vi "SCPI.vi"(4 "error in":T13, 7 "Command":string) -> (0 "error out":T13, 3 "Response":T11)   [LabVIEW 2018]
uses:
  MOKO_LabViewLibrary/MokoLowLevel/MokoLowLovelControl/MLLC_Error.ctl
  MOKO_LabViewLibrary/MokoLowLevel/MokoLowLovelControl/MLLC_Mode.ctl
  MOKO_LabViewLibrary/MokoLowLevel/MokoLowLovelControl/MLLC_Response.ctl
  MOKO_LabViewLibrary/MokoLowLevel/MokoLowLovelControl/MLLC_ConnectCluster.ctl
  MOKO_LabViewLibrary/MokoLowLevel/MokoLowLovelControl/MLLC_InterfaceType.ctl
  MOKO_LabViewLibrary/MokoLowLevel/MokoLowLovelControl/MLLC_OpenedSession.ctl
  MOKO_LabViewLibrary/MokoLowLevel/MokoLowLovelControl/MLLC_InterfaceSettings.ctl
  MOKO_LabViewLibrary/MokoLowLevel/MokoLowLovelControl/MLLC_InterfaceKind.ctl
  MOKO_LabViewLibrary/MokoLowLevel/MokoLowLovelControl/MLLC_DriverName.ctl
  MOKO_LabViewLibrary/MokoLowLevel/MokoLowLovelControl/MLLC_ErrorCode.ctl
  MOKO_LabViewLibrary/MokoLowLevel/MokoLowLovelControl/MLLC_ResponseInit.ctl
  MOKO_LabViewLibrary/MokoLowLevel/MokoLowLovelControl/MLLC_Request.ctl
panel:
  in  "Request":T1="*IDN?"
  in  "Response Init":T2="SCPI"
  in  "Error Code":T3=5450
  in  "Driver Name":T4="SCPI"
  in  "Settings":T10={"Saved Data"=variant, "Permanent data"={"Connect"={"InterfaceType"=enum."VISA", "OpenedSession"="COM1", "InterfaceSettings"={"Interface"=enum."Ethernet", "EOS 4 read"=enum."LF (\\n)", "EOS 4 write"=enum."LF (\\n)", "TMO, ms"=10000, "Sett"=variant(cluster{"Baud Rate":u32, "Data Bits":u16, "Parity":u16, "Stop Bits":u16, "Flow Control":u16, "Eho":bool} {"Baud Rate"=75, "Data Bits"=0, "Parity"=0, "Stop Bits"=0, "Flow Control"=0, "Eho"=FALSE})}}}}
  in  "Mode":T12=enum."Check"
  # "Example SCPI"
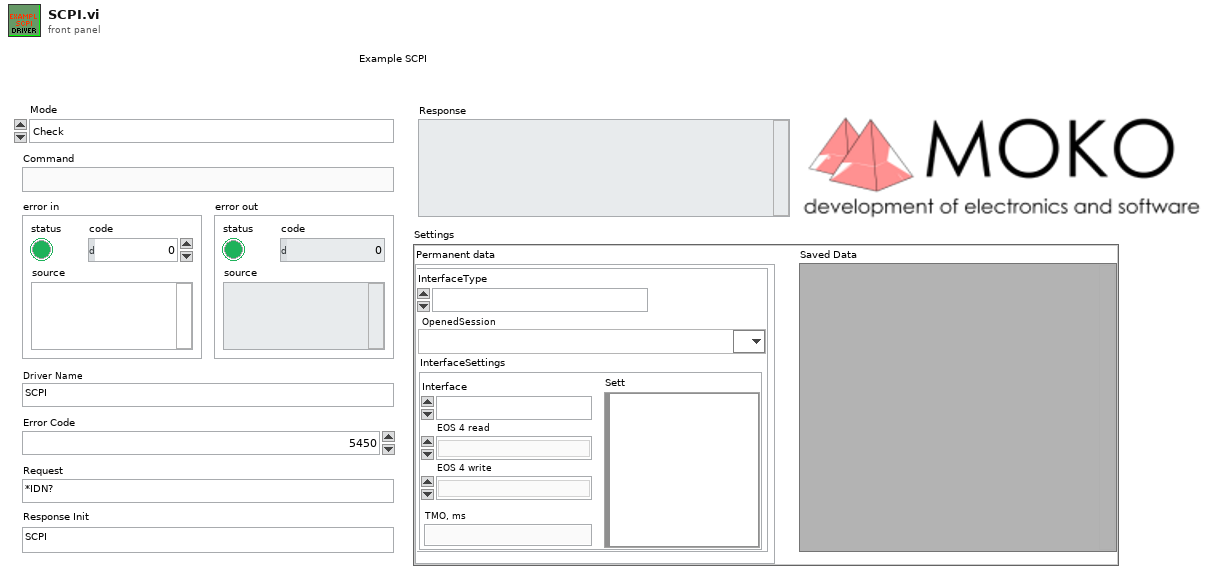
[diagram p1: front panel]
types:
  T1 = typedef "MLLC_Request.ctl" = string
  T2 = typedef "MLLC_ResponseInit.ctl" = string
  T3 = typedef "MLLC_ErrorCode.ctl" = u32
  T4 = typedef "MLLC_DriverName.ctl" = string
  T5 = typedef "MLLC_ConnectCluster.ctl" = cluster{"InterfaceType":T6, "OpenedSession":T7, "InterfaceSettings":T8}
  T6 = typedef "MLLC_InterfaceType.ctl" = enum16{"VISA", "Prologix USB-GPIB"}
  T7 = typedef "MLLC_OpenedSession.ctl" = refnum<visa-resource-name>
  T8 = typedef "MLLC_InterfaceSettings.ctl" = cluster{"Interface":T9, "EOS 4 read":enum16{"Default (=EOS 4 write)", "CR (\\r)", "LF (\\n)", "None"}, "EOS 4 write":enum16{"CR+LF (\\r\\n)", "CR (\\r)", "LF (\\n)", "None"}, "TMO, ms":i32, "Sett":variant}
  T9 = typedef "MLLC_InterfaceKind.ctl" = enum16{"RS232", "GPIB", "USB", "Ethernet", "another"}
  T10 = cluster{"Saved Data":variant, "Permanent data":cluster{"Connect":T5}}
  T11 = typedef "MLLC_Response.ctl" = string
  T12 = typedef "MLLC_Mode.ctl" = enum16{"get", "set", "close", "Init", "Check"}
  T13 = typedef "MLLC_Error.ctl" = errorcluster
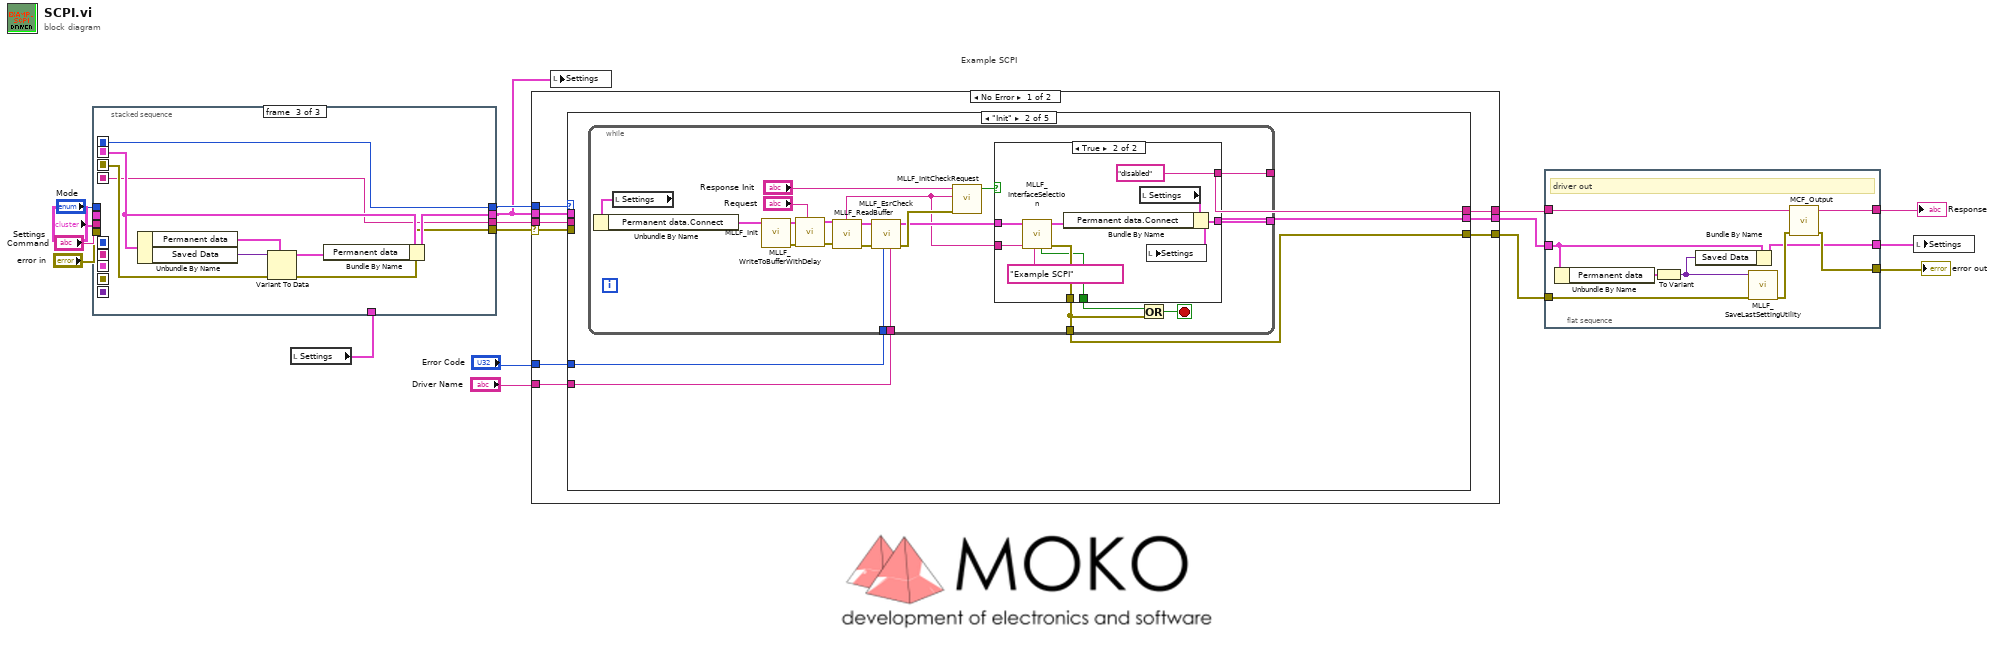
[diagram p0: block diagram]
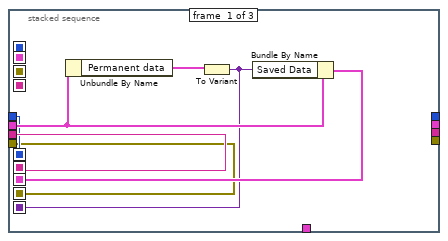
[diagram p2: hidden frame]
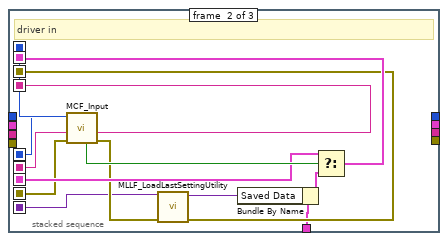
[diagram p3: hidden frame]
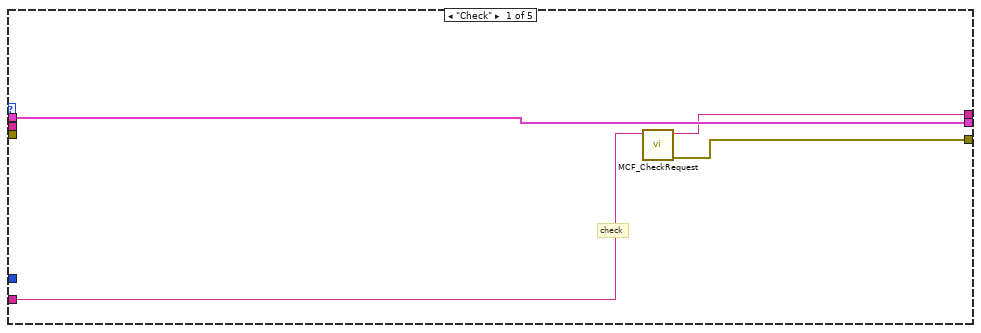
[diagram p4: hidden frame]
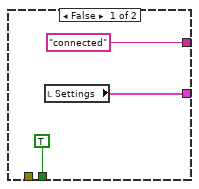
[diagram p5: hidden frame]
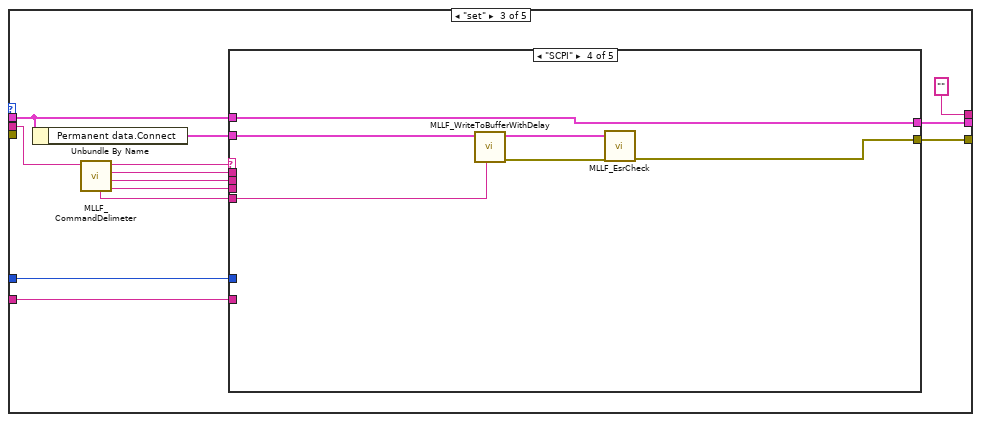
[diagram p6: hidden frame]
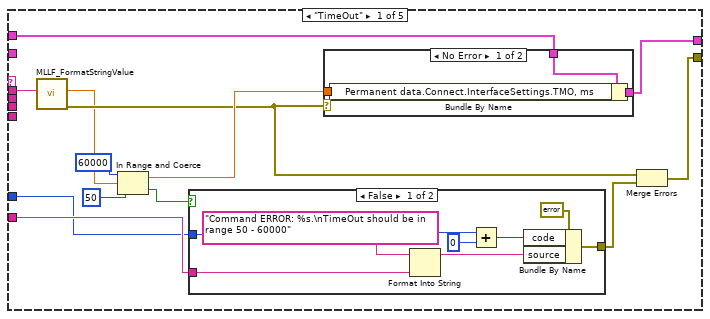
[diagram p7: hidden frame]
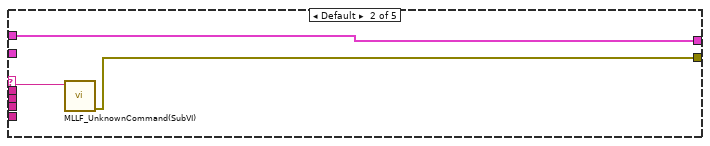
[diagram p10: hidden frame]
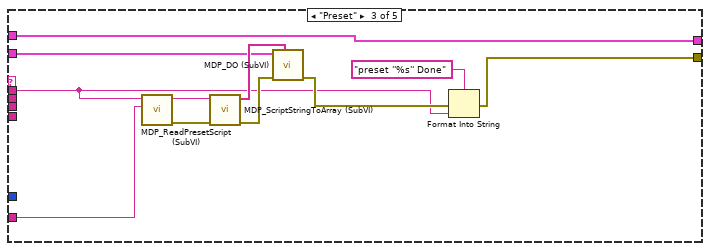
[diagram p11: hidden frame]
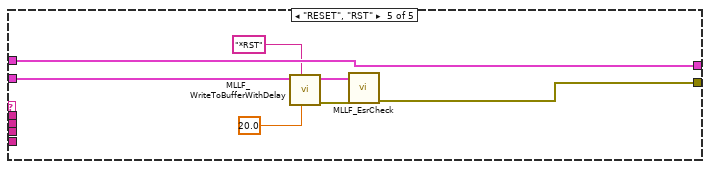
[diagram p12: hidden frame]
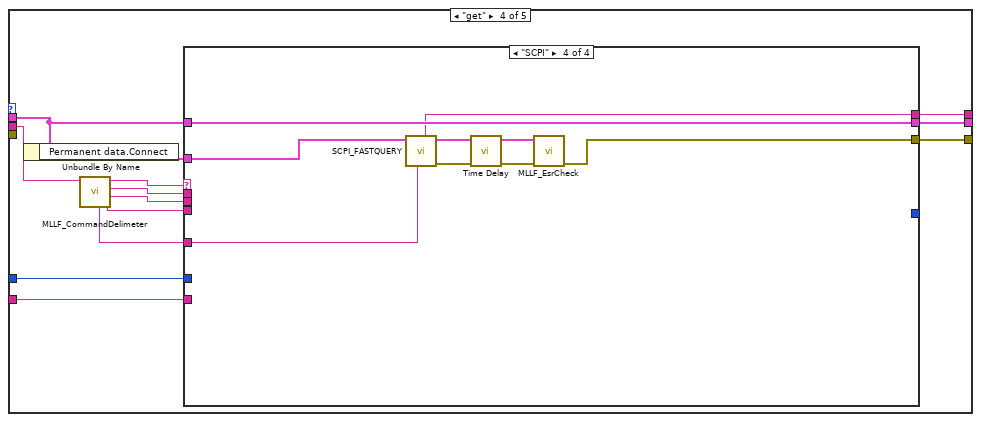
[diagram p13: hidden frame]
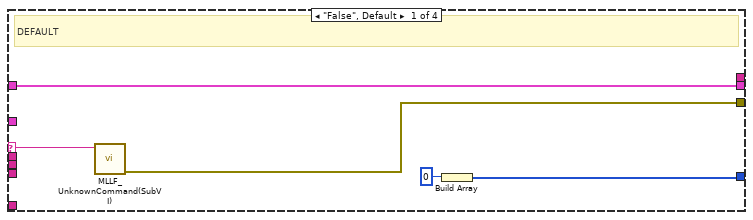
[diagram p14: hidden frame]
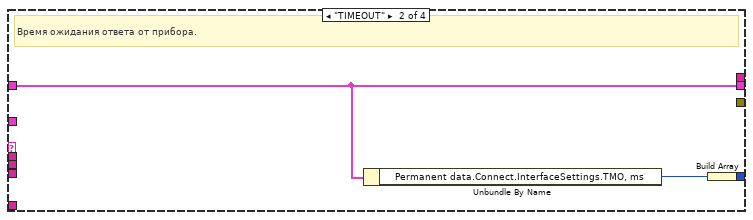
[diagram p15: hidden frame]
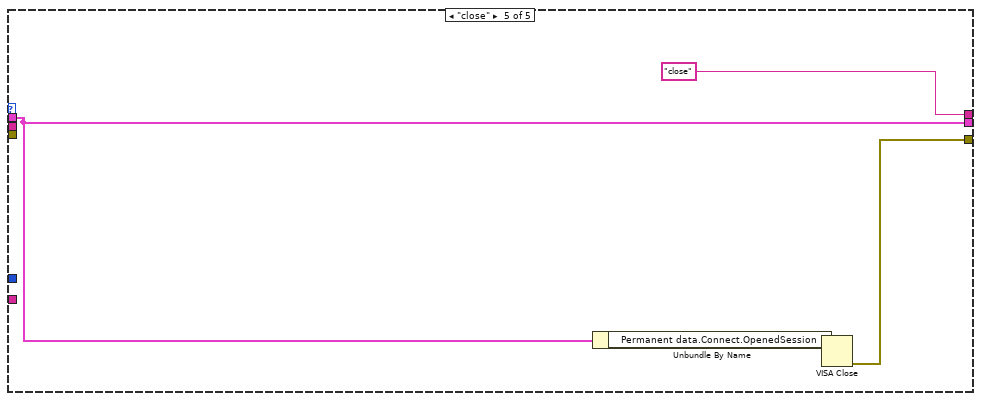
[diagram p17: hidden frame]
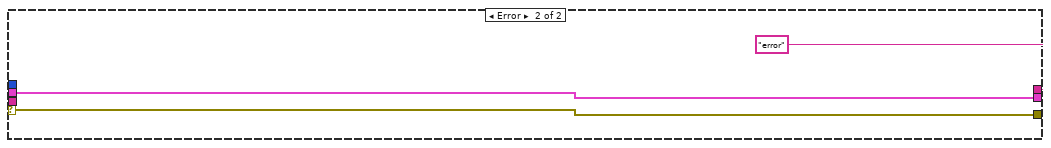
[diagram p18: hidden frame]
diagram:
  # "Example SCPI"
  n1 = local read "Settings"() -> (w7:T10)
  n2 = stacked-sequence {
    seq-local: [w20 _ _] -> [_ w36 _]
    seq-local: [w19 _ _] -> [_ w37 _]
    seq-local: [w22 _ _] -> [_ w32 _]
    seq-local: [w18 _ _] -> [_ w31 _]
    seq-local: [w21 _ _] -> [_ w27 _]
    seq-local: [_ w28 _] -> [_ _ w44]
    seq-local: [_ w38 _] -> [_ _ w41]
    seq-local: [_ w35 _] -> [_ _ w40]
    seq-local: [_ w34 _] -> [_ _ w45]
    tunnel: "Command" -> [w20 _ _]
    tunnel: "Mode" -> [w19 _ _]
    tunnel: "error in" -> [w18 _ _]
    tunnel: "Settings" -> [w23 _ _]
    tunnel: w7 -> [_ w26 _]
    tunnel: [_ _ w40] -> w9
    tunnel: [_ _ w43] -> w10
    tunnel: [_ _ w42] -> w8
    tunnel: [_ _ w41] -> w11
    frame #0 {
      n3 = Unbundle By Name(w23) -> ("Permanent data"=w24:cluster{"Connect":T5})
      n4 = To Variant(anything=w24) -> (Variant=w21:variant)
      n5 = Bundle By Name(cluster=w23, "Saved Data"=w21) -> (w22:T10)
    }
    frame #1 {
      # "driver in"
      n6 = call "MCF_Input.vi"("Error In"=w31, "Command in"=w36, "Mode in"=w37) -> ("Error Out"=w30:errorcluster, "Command out"=w35:string, "Mode out"=w38:T12, "Boolean"=w33:bool)  [unwired: 5 in]
      n7 = call "MLLF_LoadLastSettingUtility.vi"("Error In"=w30, "Save data in"=w27) -> ("Error Out"=w28:errorcluster, "Save data out"=w25:variant)  [unwired: 8 in]
      n8 = Bundle By Name(cluster=w26, "Saved Data"=w25) -> (w29:T10)
      n9 = Select(t=w32, s=w33, f=w29) -> (s? t:f=w34:T10)
    }
    frame #2 {
      n10 = Unbundle By Name(w45) -> ("Permanent data"=w46:cluster{"Connect":T5}, "Saved Data"=w39:variant)
      n11 = Variant To Data(error in=w44, type=w46, Variant=w39) -> (data=w47:cluster{"Connect":T5}, error out=w42:errorcluster)
      n12 = Bundle By Name(cluster=w45, "Permanent data"=w47) -> (w43:T10)
    }
  }
  n13 = case shown="No Error" w8 {
    selector: w8 -> [w52 w200]
    tunnel: [w54 w200] -> w4
    tunnel: w11 -> [w56 _]
    tunnel: [w55 "error" ("Output String")] -> w6
    tunnel: w9 -> [w53 _]
    tunnel: w10 -> [w49 w199]
    tunnel: "Error Code" -> [w51 _]
    tunnel: "Driver Name" -> [w50 _]
    tunnel: [w48 w199] -> w5
    frame No Error {
      n14 = case shown="\"Init\"" w56 {
        tunnel: [w58 w63 "" ("Output String") w168 "close" ("Output String")] -> w55
        tunnel: [w57 w62 w104 w170 w196] -> w54
        tunnel: w53 -> [_ _ w111 w176 _]
        tunnel: w52 -> [_ _ _ _ _]
        tunnel: w51 -> [_ w65 w110 w173 _]
        tunnel: w50 -> [w59 w64 w107 w172 _]
        tunnel: w49 -> [w60 _ w109 w175 w195]
        tunnel: [w60 w61 w108 w174 w195] -> w48
        frame "Check" {
          # "check"
          # "Проверка подленности пользователя в соответствии с протоколом MD5."
          n15 = call "MCF_CheckRequest.vi"("Driver Name"=w59) -> ("Error Out"=w57:errorcluster, "Output String"=w58:string)  [unwired: 9 in]
        }
        frame "Init" {
          # "Тут проходит инициализация оборудования"
          n16 = while {
            tunnel: [w79] -> w62
            tunnel: w65 -> [w72]
            tunnel: w64 -> [w71]
            tunnel: [w76] -> w63
            tunnel: [w77] -> w61
            stop <- w78 stop-if-true
            n17 = local read "Settings"() -> (w82:T10)
            n18 = Unbundle By Name(w82) -> ("Permanent data.Connect"=w74:T5)
            n19 = call "MLLF_Init.vi"("DriverConnect in"=w74) -> ("Error Out"=w84:errorcluster, "DriverConnect out"=w83:T5)  [unwired: 7 in]
            n20 = call "MLLF_WriteToBufferWithDelay.vi"("Command"="Request", "Error In"=w84, "DriverConnect in"=w83) -> ("Error Out"=w86:errorcluster, "DriverConnect out"=w85:T5)  [unwired: 7 in]
            n21 = call "MLLF_ReadBuffer.vi"("Error In"=w86, "DriverConnect in"=w85) -> ("Error Out"=w69:errorcluster, "DriverConnect out"=w70:T5, "String"=w66:string)  [unwired: 6 in]
            n22 = call "MLLF_EsrCheck.vi"("Name"=w71, "Error code"=w72, "error in"=w69, "DriverConnect in"=w70) -> ("error out"=w68:T13, "DriverConnect out"=w67:T5)  [unwired: 6 in]
            n23 = call "MLLF_InitCheckRequest.vi"("error in (no error)"=w68, "Answer"=w66, "Response Init"="Response Init") -> ("Design"=w73:bool)  [unwired: 5 in, 3 out]
            n24 = case shown="True" w73 {
              tunnel: w67 -> [_ w97]
              tunnel: [TRUE w91] -> w80
              tunnel: [_ w98] -> w79
              tunnel: [w88 w93] -> w77
              tunnel: ["connected" "disabled"] -> w76
              tunnel: w66 -> [_ w90]
              frame False {
                n25 = local read "Settings"() -> (w88:T10)
              }
              frame True {
                n26 = call "MLLF_InterfaceSelection.vi"("Driver Name"="Example SCPI" ("String"), "Answer:"=w90, "DriverConnect in"=w97) -> ("error out"=w98:T13, "DriverConnect out"=w95:T5, "stop init?"=w91:bool)  [unwired: 4 in, 2 out]
                n27 = local read "Settings"() -> (w94:T10)
                n28 = Bundle By Name(cluster=w94, "Permanent data.Connect"=w95) -> (w93:T10)
                n29 = local write "Settings"(w93) -> ()
              }
            }
            n30 = Or(x=w80, y=w79) -> (x .or. y?=w78:bool)
          }
        }
        frame "set" {
          # "Тут реализованы функции DriverSet"
          n31 = Unbundle By Name(w109) -> ("Permanent data.Connect"=w105:T5)
          n32 = call "MLLF_CommandDelimeter.vi"("command with param"=w111) -> ("param 3"=w100:string, "param 2"=w101:string, "param 1"=w102:string, "command"=w103:string, "Spit delimetre"=w99:string)  [unwired: 6 in]
          n33 = case shown="\"SCPI\"" w103 {
            selector: w103 -> [_ w138 _ _ _]
            tunnel: w109 -> [w114 w139 w140 w155 w163]
            tunnel: [w113 w139 w140 w155 w163] -> w108
            tunnel: w102 -> [w112 _ w143 _ _]
            tunnel: w110 -> [w116 _ _ _ _]
            tunnel: w107 -> [w117 _ w142 _ _]
            tunnel: [w115 w137 w141 w154 w162] -> w104
            tunnel: w105 -> [_ _ w144 w156 w161]
            tunnel: w101 -> [_ _ _ _ _]
            tunnel: w100 -> [_ _ _ _ _]
            tunnel: w99 -> [_ _ _ w151 _]
            frame "TimeOut" {
              n34 = call "MLLF_FormatStringValue.vi"("String Value"=w112) -> ("error out"=w119:T13, "number"=w118:dbl)  [unwired: 8 in, 1 out]
              n35 = In Range and Coerce(upper limit=60000, x=w118, lower limit=50) -> (coerced(x)=w122:dbl, In Range?=w120:bool)
              n36 = case shown="False" w120 {
                tunnel: [w131 _] -> w121
                tunnel: w116 -> [w130 _]
                tunnel: w117 -> [w129 _]
                frame False {
                  n37 = Format Into String(format string="Command ERROR: %s.\nTimeOut should be in range 50 - 60000", w129) -> (resulting string=w133:string)  [unwired: 2 in, 1 out]
                  n38 = Add(x=w130, y=0) -> (x+y=w134:T3)
                  n39 = Bundle By Name(cluster=errorcluster {"status"=TRUE, "code"=0, "source"=""} ("error out"), "code"=w134, "source"=w133) -> (w131:errorcluster)
                }
                frame True {
                }
              }
              n40 = case shown="No Error" w119 {
                tunnel: [w127 w128] -> w113
                tunnel: w114 -> [w126 w128]
                tunnel: w122 -> [w125 _]
                frame No Error {
                  n41 = Bundle By Name(cluster=w126, "Permanent data.Connect.InterfaceSettings.TMO, ms"=w125) -> (w127:T10)
                }
                frame Error {
                }
              }
              n42 = Merge Errors(w119, w121) -> (w115:errorcluster)
            }
            frame Default {
              n43 = call "MLLF_UnknownCommand(SubVI).vi"("Unknown command"=w138) -> ("error out"=w137:errorcluster)  [unwired: 10 in]
            }
            frame "Preset" {
              n44 = call "MDP_ReadPresetScript (SubVI).vi"("Driver Name"=w142, "String in"=w143) -> ("Error Out"=w148:errorcluster, "String out"=w149:string)  [unwired: 8 in]
              n45 = call "MDP_ScriptStringToArray (SubVI).vi"("Error In"=w148, "String script"=w149) -> ("Error Out"=w150:errorcluster, "Array script"=w145:string[])  [unwired: 8 in]
              n46 = call "MDP_DO (SubVI).vi"("Array script"=w145, "Error in (no error)"=w150, "DriverConnect in"=w144) -> ("Error Out"=w146:errorcluster)  [unwired: 7 in, 1 out]
              n47 = Format Into String(format string="preset ''%s'' Done" ("Befor substring"), error in=w146, w143) -> (error out=w141:errorcluster)  [unwired: 1 in, 1 out]
            }
            frame "SCPI" {
              n48 = call "MLLF_WriteToBufferWithDelay.vi"("Command"=w151, "DriverConnect in"=w156) -> ("Error Out"=w152:errorcluster, "DriverConnect out"=w153:T5)  [unwired: 8 in]
              n49 = call "MLLF_EsrCheck.vi"("error in"=w152, "DriverConnect in"=w153) -> ("error out"=w154:T13)  [unwired: 8 in, 1 out]
            }
            frame "RESET", "RST" {
              n50 = call "MLLF_WriteToBufferWithDelay.vi"("Delay Time ( 0,05 s)"=20.0, "Command"="*RST" ("string"), "DriverConnect in"=w161) -> ("Error Out"=w159:errorcluster, "DriverConnect out"=w158:T5)  [unwired: 7 in]
              n51 = call "MLLF_EsrCheck.vi"("error in"=w159, "DriverConnect in"=w158) -> ("error out"=w162:T13)  [unwired: 8 in, 1 out]
            }
          }
        }
        frame "get" {
          # "Тут реализованы функции DriverGet"
          n52 = Unbundle By Name(w175) -> ("Permanent data.Connect"=w171:T5)
          n53 = call "MLLF_CommandDelimeter.vi"("command with param"=w176) -> ("param 3"=w165:string, "param 2"=w166:string, "param 1"=w167:string, "command"=w169:string, "Spit delimetre"=w164:string)  [unwired: 6 in]
          n54 = case shown="\"SCPI\"" w169 {
            selector: w169 -> [w178 _ _ _]
            tunnel: [w177 _ _ w190] -> w170
            tunnel: w173 -> [_ _ _ _]
            tunnel: [w181 w184 w185 w192] -> w174
            tunnel: w175 -> [w181 w184 w185 w192]
            tunnel: [w179 w182 _ _] -> _
            tunnel: w171 -> [_ _ _ w193]
            tunnel: w172 -> [_ _ _ _]
            tunnel: [_ _ _ w189] -> w168
            tunnel: w167 -> [_ _ _ _]
            tunnel: w166 -> [_ _ _ _]
            tunnel: w165 -> [_ _ _ _]
            tunnel: w164 -> [_ _ _ w186]
            frame "False", Default {
              # "DEFAULT"
              n55 = call "MLLF_UnknownCommand(SubVI).vi"("Unknown command"=w178) -> ("error out"=w177:errorcluster)  [unwired: 10 in]
              n56 = Build Array(0 ("TimeOut")) -> (w179:i32[])
            }
            frame "TIMEOUT" {
              # "Время ожидания ответа от прибора."
              n57 = Unbundle By Name(w184) -> ("Permanent data.Connect.InterfaceSettings.TMO, ms"=w183:i32)
              n58 = Build Array(w183) -> (w182:i32[])
            }
            frame "------ID-------" {
            }
            frame "SCPI" {
              n59 = call "SCPI_FASTQUERY.vi"("input"=w186, "DriverConnect in"=w193) -> ("error out"=w188:T13, "DriverConnect out"=w191:T5, "output"=w189:string)  [unwired: 7 in]
              n60 = call "Time Delay"("error in (no error)"=w188) -> ("error out"=w187:errorcluster)  [unwired: 10 in]
              n61 = call "MLLF_EsrCheck.vi"("error in"=w187, "DriverConnect in"=w191) -> ("error out"=w190:T13)  [unwired: 8 in, 1 out]
            }
          }
        }
        frame "close" {
          # "Завершение сессии"
          n62 = Unbundle By Name(w195) -> ("Permanent data.Connect.OpenedSession"=w197:T7)
          n63 = VISA Close(VISA resource name=w197) -> (error out=w196:errorcluster)  [unwired: 1 in]
        }
      }
    }
    frame Error {
    }
  }
  n64 = local write "Settings"(w10) -> ()
  n65 = flat-sequence {
    tunnel: [w209] -> w3
    tunnel: [w208] -> w2
    tunnel: w6 -> [w207]
    tunnel: w4 -> [w206]
    tunnel: w5 -> [w202]
    tunnel: [w204] -> w1
    frame #0 {
      # "driver out"
      n66 = Unbundle By Name(w202) -> ("Permanent data"=w201:cluster{"Connect":T5})
      n67 = To Variant(anything=w201) -> (Variant=w203:variant)
      n68 = Bundle By Name(cluster=w202, "Saved Data"=w203) -> (w204:T10)
      n69 = call "MLLF_SaveLastSettingUtility.vi"("error in"=w206, "Saved Data"=w203) -> ("error out"=w205:T13)  [unwired: 8 in, 1 out]
      n70 = call "MCF_Output.vi"("Error In"=w205, "Input"=w207) -> ("Error Out"=w208:errorcluster, "Output"=w209:string)  [unwired: 8 in]
    }
  }
  n71 = local write "Settings"(w1) -> ()
  "error out" <- w2
  "Response" <- w3
